vi "Test CameraTool Focus.vi"() -> ()   [LabVIEW 2011]
uses:
  CameraTool Class.lvclass
  Vec3d Class/Vec3d Class.lvclass
  Gantry Class/Gantry Class.lvclass
panel:
  out "Focus Routine Running":bool
  in  "HOME?":bool
  in  "Config Folder":path=path "C:/Users/Husker/Desktop/gantry/Config"
  out "error out":errorcluster
  out "start_focus_height":dbl
  out "measured_focus_height":sgl
  in  "stop":bool
  in  "Find Focus":bool
  out "Image Preview":T1(plugin-control)
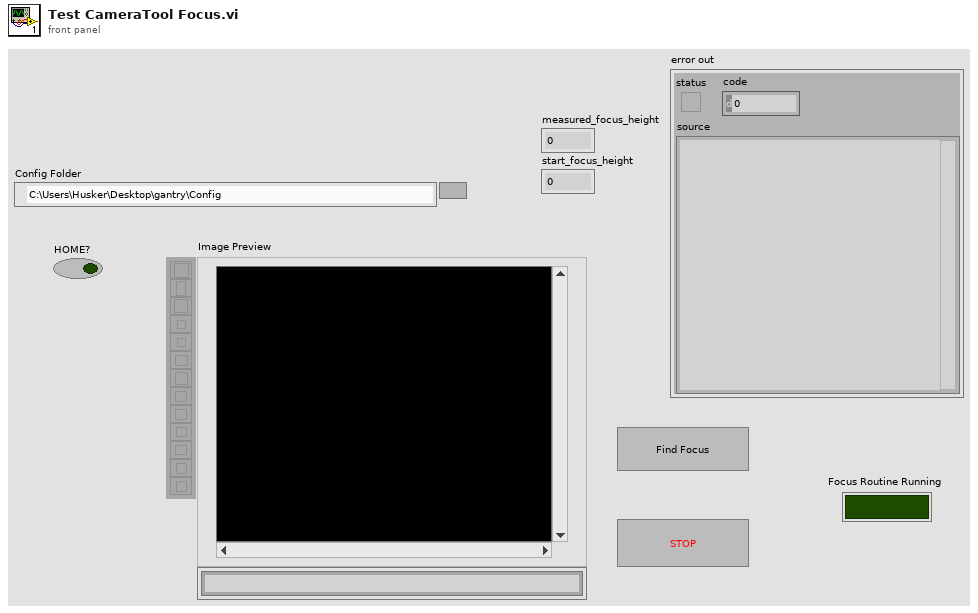
[diagram p1: front panel]
types:
  T1 = typedef "IMAQ Image.ctl" = refnum<image>
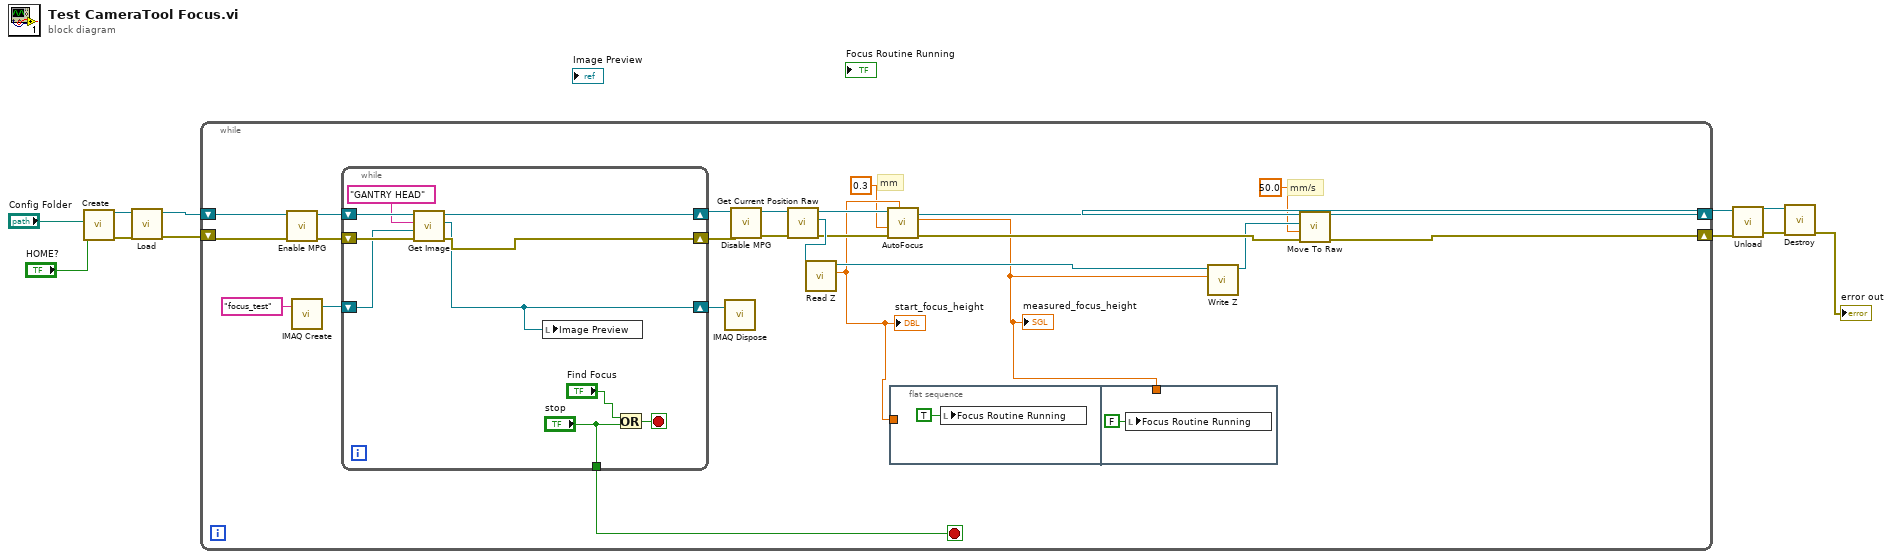
[diagram p0: block diagram]
diagram:
  n1 = call "Create.vi"("HOME?"="HOME?", "Config Folder"="Config Folder") -> ("error out"=w10:errorcluster, "Gantry out"=w11:refnum<class "Gantry Class.lvclass">)  [unwired: 8 in]
  n2 = call "Load.vi"("error in"=w10, "Gantry In"=w11) -> ("error out"=w8:errorcluster, "CameraTool out"=w9:refnum<class "CameraTool Class.lvclass">)  [unwired: 8 in]
  n3 = while {
    shift-right: [w30] -> w7
    shift-left: w9 -> [w18]
    shift-right: [w29] -> w6
    shift-left: w8 -> [w15]
    stop <- w12 stop-if-true
    # "mm"
    # "mm/s"
    n4 = call-dynamic "Enable MPG.vi"("error in (no error)"=w15, "Gantry Class in"=w18) -> ("error out"=w16:errorcluster, "Gantry Class out"=w17:refnum<class "CameraTool Class.lvclass">)  [unwired: 8 in]
    n5 = call "IMAQ Create"("Image Name"="focus_test") -> ("New Image"=w24:T1)  [unwired: 4 in, 1 out]
    n6 = while {
      shift-right: [w47] -> w22
      shift-left: w17 -> [w48]
      shift-right: [w43] -> w20
      shift-left: w16 -> [w46]
      shift-right: [w42] -> w23
      shift-left: w24 -> [w40]
      tunnel: ["stop"] -> w12
      stop <- w44 stop-if-true
      n7 = call-dynamic "Get Image.vi"("error in"=w46, "Image In"=w40, "Camera Name"="GANTRY HEAD", "Gantry in"=w48) -> ("error out"=w43:errorcluster, "Image Out"=w42:T1, "Gantry out"=w47:refnum<class "CameraTool Class.lvclass">)  [unwired: 5 in]
      n8 = local write "Image Preview"(w42) -> ()
      n9 = Or(x="Find Focus", y="stop") -> (x .or. y?=w44:bool)
    }
    n10 = call "IMAQ Dispose"("Image"=w23) -> ()  [unwired: 5 in, 1 out]
    n11 = call-dynamic "Disable MPG.vi"("error in (no error)"=w20, "Gantry Class in"=w22) -> ("error out"=w19:errorcluster, "Gantry Class out"=w21:refnum<class "CameraTool Class.lvclass">)  [unwired: 8 in]
    n12 = call-dynamic "Get Current Position Raw.vi"("error in (no error)"=w19, "Gantry Class in"=w21) -> ("error out"=w35:errorcluster, "Vec3d Class out"=w36:refnum<class "Vec3d Class.lvclass">, "Gantry Class out"=w28:refnum<class "CameraTool Class.lvclass">)  [unwired: 7 in]
    n13 = call-dynamic "Read Z.vi"("Vec3d Class in"=w36) -> ("Z"=w26:dbl, "Vec3d Class out"=w33:refnum<class "Vec3d Class.lvclass">)  [unwired: 8 in, 1 out]
    "start_focus_height" <- w26
    n14 = call-dynamic "AutoFocus.vi"("Start Z"=w26, "error in"=w35, "Range"=0.3, "CameraTool Class In"=w28) -> ("error out"=w34:errorcluster, "focus height"=w32:sgl, "CameraTool Class Out"=w27:refnum<class "CameraTool Class.lvclass">)  [unwired: 5 in]
    "measured_focus_height" <- w32
    n15 = flat-sequence {
      tunnel: w26 -> [_]
      tunnel: w32 -> [_]
      frame #0 {
        n16 = local write "Focus Routine Running"(TRUE ("Focus Routine Running")) -> ()
      }
      frame #1 {
        n17 = local write "Focus Routine Running"(FALSE ("Focus Routine Running")) -> ()
      }
    }
    n18 = call-dynamic "Write Z.vi"("Z"=w32, "Vec3d Class in"=w33) -> ("Vec3d Class out"=w31:refnum<class "Vec3d Class.lvclass">)  [unwired: 8 in, 1 out]
    n19 = call-dynamic "Move To Raw.vi"("error in"=w34, "Speed"=50.0, "Destination"=w31, "Gantry in"=w27) -> ("error out"=w29:errorcluster, "Gantry out"=w30:refnum<class "CameraTool Class.lvclass">)  [unwired: 6 in]
  }
  n20 = call "Unload.vi"("error in (no error)"=w6, "CameraTool in"=w7) -> ("error out"=w4:errorcluster, "Gantry out"=w5:refnum<class "Gantry Class.lvclass">)  [unwired: 8 in]
  n21 = call "Destroy.vi"("error in"=w4, "Gantry Class in"=w5) -> ("error out"=→"error out":errorcluster)  [unwired: 9 in]
